vi "Read States.vi"(8 "error in (no error)":errorcluster, 11 "DefendGoalTactic in":refnum<class "DefendGoalTactic.lvclass">) -> (0 "error out":errorcluster, 2 "States":T1, 3 "DefendGoalTactic out":refnum<class "DefendGoalTactic.lvclass">)   [LabVIEW 2024, in "DefendGoalTactic.lvclass"]
uses:
  DefendGoalTactic.lvclass
  DefendGoalTacticStates.ctl
  DefendGoalTactic.lvclass/DefendGoalTactic.ctl
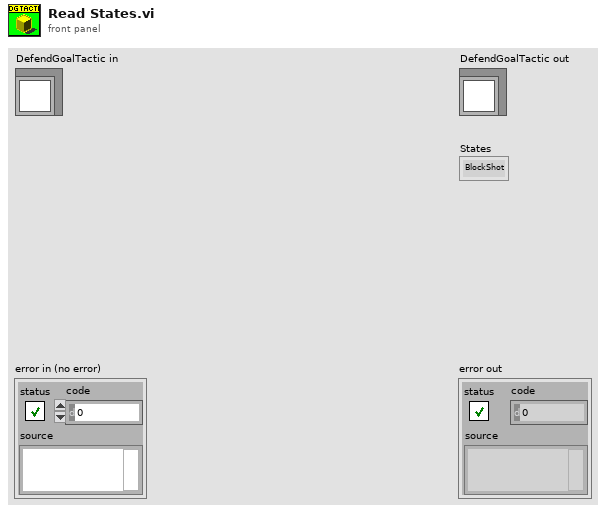
[diagram p1: front panel]
types:
  T1 = typedef "DefendGoalTactic.lvclass/DefendGoalTacticStates.ctl" = enum16{"BlockShot", "BlockPossibleShot", "CoverOneTouchShot", "Kick", "GuardGoal", "Exit"}
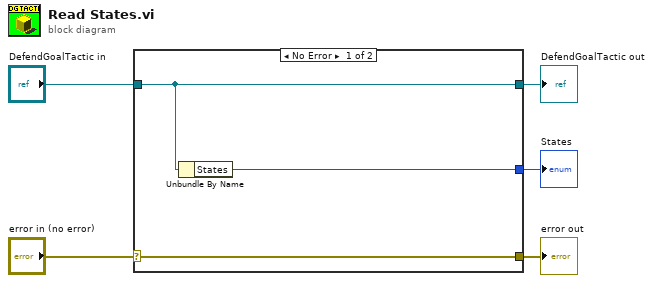
[diagram p0: block diagram]
diagram:
  n1 = case shown="No Error" "error in (no error)" {
    selector: "error in (no error)" -> [w8 w9]
    tunnel: [w8 w9] -> w4
    tunnel: [w7 w10] -> w2
    tunnel: "DefendGoalTactic in" -> [w7 w10]
    tunnel: [w6 _] -> w1
    frame No Error {
      n2 = Unbundle By Name(w7) -> ("States"=w6:T1)
    }
    frame Error {
    }
  }
  "error out" <- w4
  "DefendGoalTactic out" <- w2
  "States" <- w1
